vi "SRV_PM_Evaluate Packet Data.vi"(0 "Packet Data":u8[](array[numeric]) format="%.0x", 11 "error in (no error)":errorcluster) -> (4 "Packet Data dup":u8[](array[numeric]) format="%.0x", 8 "Packet":T1 {"Packet Data" format="%.0x"}, 10 "Packet Complete?":bool, 14 "Extra Bytes":u8[](array[numeric]) format="%.0x", 15 "error out":errorcluster)   [LabVIEW 2009]
uses:
  SRV_PM_Packet.ctl
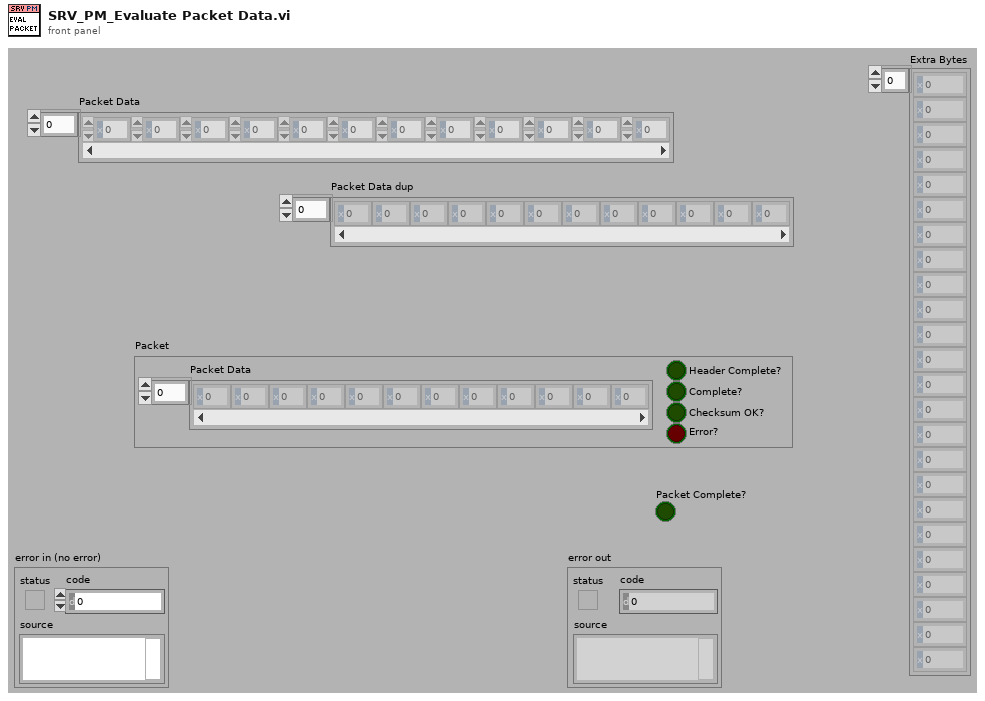
[diagram p1: front panel]
types:
  T1 = typedef "SRV_PM_Packet.ctl" = cluster{"Packet Data":u8[], "Header Complete?":bool, "Complete?":bool, "Checksum OK?":bool, "Error?":bool}
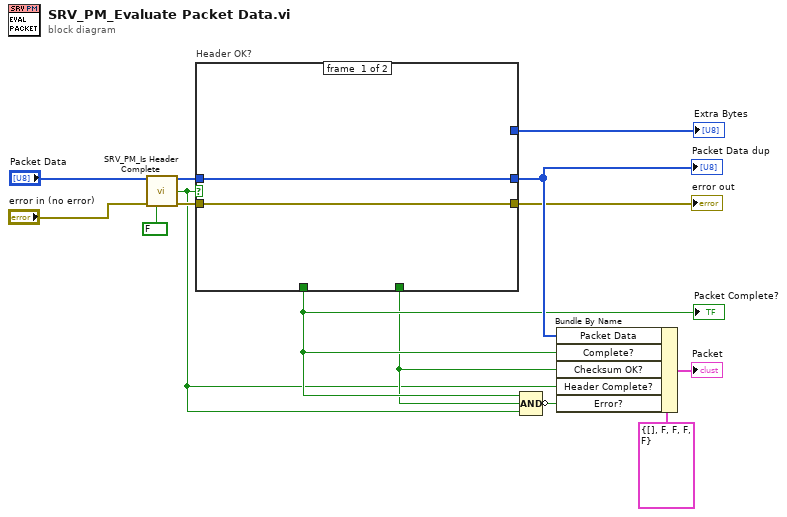
[diagram p0: block diagram]
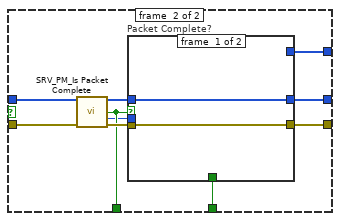
[diagram p2: hidden frame]
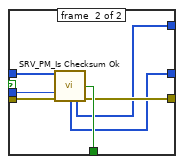
[diagram p3: hidden frame]
diagram:
  n1 = call "SRV_PM_Is Header Complete.vi"("Packet Data"="Packet Data", "error in (no error)"="error in (no error)", "Gen Err? (T)"=FALSE) -> ("Packet Data dup"=w12:u8[], "Header OK?"=w2:bool, "error out"=w11:errorcluster)  [unwired: 10 in]
  n2 = case "Header OK?" shown="True" w2 {
    tunnel: w12 -> [w16 w19]
    tunnel: w11 -> [w15 w18]
    tunnel: [w16 w22] -> w9
    tunnel: [_ w21] -> w8
    tunnel: [_ w26] -> w7
    tunnel: [w15 w23] -> w5
    tunnel: [_ w20] -> w1
    frame #0 {
    }
    frame #1 {
      n3 = call "SRV_PM_Is Packet Complete.vi"("Packet Data"=w19, "error in (no error)"=w18) -> ("Packet Data dup"=w25:u8[], "Packet Complete?"=w21:bool, "Total Packet Length"=w17:u16, "error out"=w24:errorcluster)  [unwired: 10 in]
      n4 = case "Packet Complete?" shown="True" w21 {
        tunnel: [_ w35] -> w26
        tunnel: w25 -> [w28 w34]
        tunnel: w24 -> [w27 w33]
        tunnel: [w27 w32] -> w23
        tunnel: [w28 w31] -> w22
        tunnel: [_ w30] -> w20
        tunnel: w17 -> [_ w29]
        frame #0 {
        }
        frame #1 {
          n5 = call "SRV_PM_Is Checksum Ok.vi"("Packet Data"=w34, "Total Packet Length"=w29, "error in (no error)"=w33) -> ("Checksum OK?"=w35:bool, "Packet Data sans Extra Bytes"=w31:u8[], "Extra Bytes"=w30:u8[], "error out"=w32:errorcluster)  [unwired: 9 in]
        }
      }
    }
  }
  "Packet Data dup" <- w9
  "error out" <- w5
  "Packet Complete?" <- w8
  "Extra Bytes" <- w1
  n6 = Compound Arithmetic op=AND(w8, w7, w2) -> (invert w6:bool)
  n7 = Bundle By Name(cluster=T1 {"Packet Data"=[], "Header Complete?"=FALSE, "Complete?"=FALSE, "Checksum OK?"=FALSE, "Error?"=FALSE} ("Packet"), "Packet Data"=w9, "Complete?"=w8, "Checksum OK?"=w7, "Header Complete?"=w2, "Error?"=w6) -> (→"Packet":T1)
